vi "DSF.Engine.Plugin.Set Iteration.vi"(11 "Plugin in":refnum<class "DSF.Engine.Plugin.lvclass">) -> (3 "Plugin out":refnum<class "DSF.Engine.Plugin.lvclass">)   [LabVIEW 2017, in "DSF.Engine.lvlib" / "DSF.Engine.Plugin.lvclass"]
uses:
  DSF.Engine.Plugin.lvclass
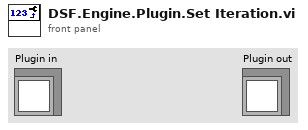
[diagram p1: front panel]
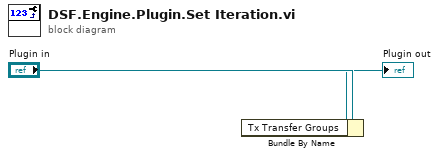
[diagram p0: block diagram]
diagram:
  n1 = Bundle By Name(cluster="Plugin in") -> (→"Plugin out":refnum<class "DSF.Engine.Plugin.lvclass">)  [unwired: 1 in]
